vi "HIA.vi"(0 "System no.":i32=1 min=1 max=4 step=1, 2 "Axis to set":string[](array[string]), 3 "DeviceID":i32[](array[numeric]), 5 "error in":errorcluster, 6 "Function":i32[](array[numeric]), 10 "DeviceAxis":i32[](array[numeric])) -> (14 "Controller error":bool, 19 "error out":errorcluster)   [LabVIEW 2020]
doc: "This VI assigns an axis of a Human Interface Device (HID) to a function of a controller axis. Human interface device control must be disabled (HIN command) when you change HIA. If DeviceID and DeviceAxis is 0, the function is deactivated. See controller user manual for details.\nThe VI waits 100 ms and queries ERR?. Controller error is TRUE if selected system reports error code which is not equal to 0.\n\nC-867: The configuration with HIA is done in volatile memory only (RAM). Use WPA to save the current configuration to non-volatile memory. See controller user manual for details.\n\nC-884, E-871, E-872, E-873: The configuration with HIA is done in volatile memory only (RAM). Use WPA to save the current configuration to non-volatile memory. See controller user manual for details."
panel:
  # "This vi assigns a HID axis to a function of a controller axis. Human interface device control must be \ndisabled (command HIN) when you change HIA. If DeviceID and DeviceAxis is 0, the function is deactivated\nThe VI waits 100 ms and queries ERR?. See controller User Manual for details. Controller error is TRUE if \nselected system reports error code not equal to 0."
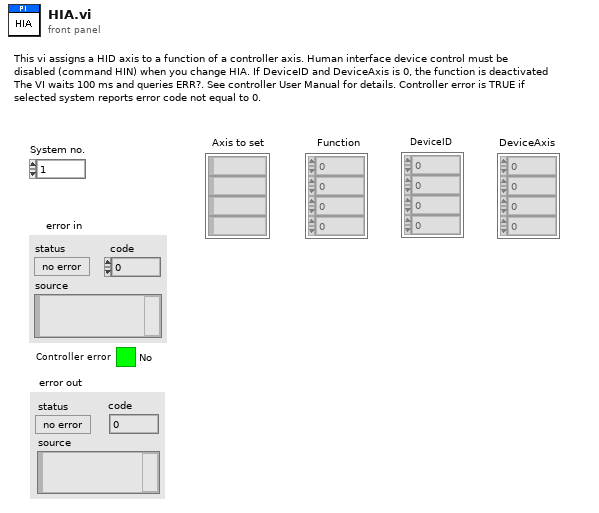
[diagram p1: front panel]
types:
  T1 = enum16{"Disable error check", "Force error check", "Use global settings"}
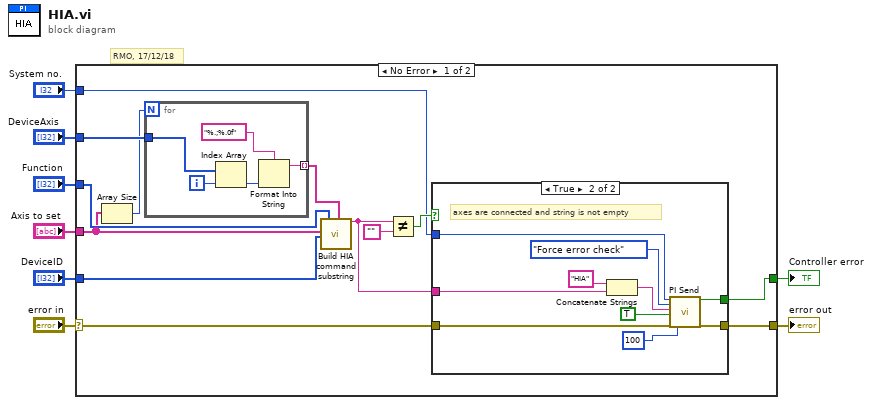
[diagram p0: block diagram]
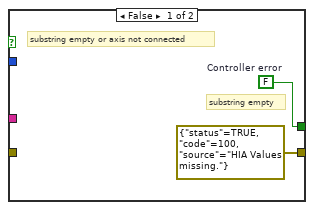
[diagram p2: hidden frame]
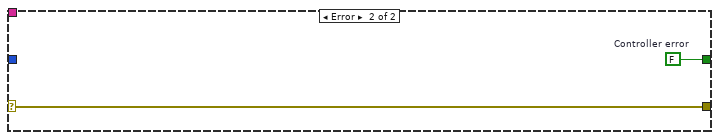
[diagram p3: hidden frame]
diagram:
  # "RMO, 17/12/18"
  n1 = case shown="No Error" "error in" {
    selector: "error in" -> [w10 w40]
    tunnel: [w21 w40] -> w8
    tunnel: "DeviceID" -> [w18 _]
    tunnel: "System no." -> [w15 _]
    tunnel: "Axis to set" -> [w13 _]
    tunnel: "Function" -> [w17 _]
    tunnel: "DeviceAxis" -> [w14 _]
    tunnel: [w9 w39] -> w1
    frame No Error {
      n2 = Array Size(array=w13) -> (size(s)=w12:i32)
      n3 = for {
        N: w12 -> [_]
        tunnel: w14 -> [w25]
        tunnel: [w22] -> w11 mode=indexing
        i -> [w24]
        n4 = Index Array(array=w25, index=w24) -> (element=w23:i32)
        n5 = Format Into String(format string="%.;%.0f" ("Format String"), w23) -> (resulting string=w22:string)  [unwired: 2 in, 1 out]
      }
      n6 = call "Build HIA command substring.vi"("Axes to set"=w13, "DeviceID"=w18, "Function"=w17, "DeviceAxis"=w11) -> ("HIA command substring"=w19:string)  [unwired: 1 in, 14 out]
      n7 = Not Equal?(x=w19, y="") -> (x != y?=w16:bool)
      n8 = case shown="True" w16 {
        tunnel: w19 -> [_ w37]
        tunnel: [errorcluster {"status"=TRUE, "code"=100, "source"="HIA Values missing."} ("error out") w30] -> w21
        tunnel: w10 -> [_ w34]
        tunnel: w15 -> [_ w33]
        tunnel: [w27 w29] -> w9
        frame False {
          w27 = FALSE  # Controller error
          # "substring empty"
          # "substring empty or axis not connected"
        }
        frame True {
          # "axes are connected and string is not empty"
          n9 = Concatenate Strings("HIA", w37) -> (w35:string)
          n10 = call "PI Send.vi"("System no."=w33, "Error check settings"=T1."Force error check", "String to send"=w35, "Attach termination char.?"=TRUE ("Attach Linefeed?"), "error in"=w34, "Delay before error check (ms)"=u32 100 ("milliseconds to wait")) -> ("Controller error"=w29:bool, "error out"=w30:errorcluster)  [unwired: 12 out]
        }
      }
    }
    frame Error {
      w39 = FALSE  # Controller error
    }
  }
  "error out" <- w8
  "Controller error" <- w1
